vi "Close RS422A.vi"(4 "Source (\"\")":string, 6 "Timeout (25000)":u32=25000, 8 "error in (no error)":errorcluster, 10 "Address (1)":i32=1 min=1 max=99 step=1, 11 "VISA resource name":refnum<visa-resource-name>) -> (0 "error out":errorcluster, 3 "VISA resource name out":refnum<visa-resource-name>)   [LabVIEW 2020, in "Yokogawa GX Series.lvlib"]
doc: "Closes RS-422A/485."
uses:
  <instrlib>/Yokogawa GX Series/Yokogawa GX Series.lvlib
panel:
  # "msec"
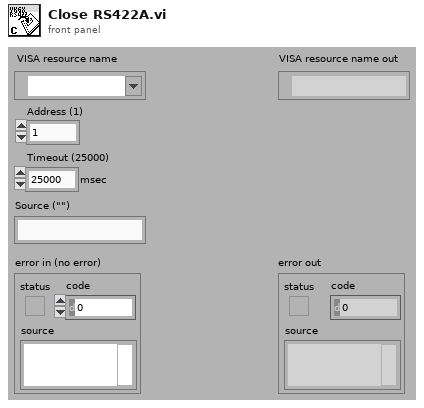
[diagram p1: front panel]
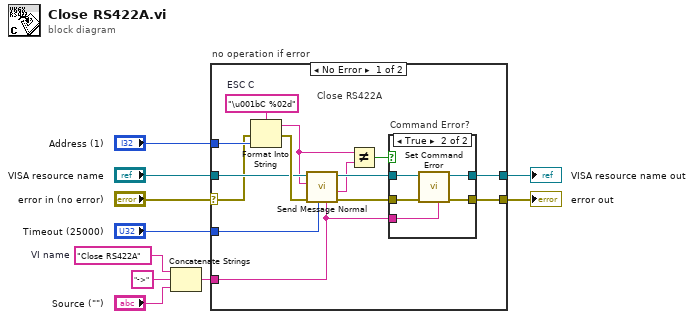
[diagram p0: block diagram]
diagram:
  w5 = "Close RS422A"  # VI name
  n1 = Concatenate Strings(w5, "->", "Source (\"\")") -> (w2:string)
  n2 = case "no operation if error" shown="No Error" "error in (no error)" {
    selector: "error in (no error)" -> [w11 w32]
    tunnel: "Address (1)" -> [w24 _]
    tunnel: "VISA resource name" -> [w13 w33]
    tunnel: [w22 w33] -> w9
    tunnel: [w21 w32] -> w8
    tunnel: "Timeout (25000)" -> [w15 _]
    tunnel: w2 -> [w16 _]
    frame No Error {
      w23 = "\u001bC %02d"  # ESC C
      # "Close RS422A"
      n3 = Format Into String(format string=w23, error in=w11, w24) -> (resulting string=w12:string, error out=w14:errorcluster)  [unwired: 1 in]
      n4 = call <instrlib>:"Send Message Normal.vi"("Source (\"\")"=w16, "Timeout (25000)"=w15, "error in (no error)"=w14, "Send Message (\"\")"=w12, "VISA resource name"=w13) -> ("error out"=w19:errorcluster, "Read Buffer"=w17:string, "VISA resource name out"=w18:refnum<visa-resource-name>)  [unwired: 4 out]
      n5 = Not Equal?(x=w12, y=w17) -> (x != y?=w20:bool)
      n6 = case "Command Error?" shown="True" w20 {
        tunnel: w18 -> [w26 w31]
        tunnel: w19 -> [w25 w30]
        tunnel: [w26 w29] -> w22
        tunnel: [w25 w27] -> w21
        tunnel: w16 -> [_ w28]
        frame False {
        }
        frame True {
          n7 = call <instrlib>:"Set Command Error.vi"("Source (\"\")"=w28, "error in (no error)"=w30, "VISA resource name"=w31) -> ("error out"=w27:errorcluster, "VISA resource name out"=w29:refnum<visa-resource-name>)  [unwired: 7 out]
        }
      }
    }
    frame Error {
    }
  }
  "VISA resource name out" <- w9
  "error out" <- w8
